vi "ArduinoLib.vi"() -> ()   [LabVIEW 2020]
uses:
  <vilib>/LabVIEW Interface for Arduino/Type Defs/Board Type.ctl
  <vilib>/LabVIEW Interface for Arduino/Type Defs/Connection Type.ctl
  <vilib>/LabVIEW Interface for Arduino/LabVIEW Interface for Arduino.lvlib
panel:
  in  "Connection Type (USB/Serial)":T1
  in  "Bytes Per Packet (15)":u32=15
  in  "milliseconds to wait":u32
  in  "Time Out (100 ms)":i32=100
  in  "Bytes To Read (0)":u8
  out "Read Buffer":string
  in  "stop":bool
  out "error out":errorcluster
  in  "error in (no error)":errorcluster
  in  "Board Type (Uno)":T2
  in  "Baud Rate (115200)":u32=115200
  in  "VISA resource":refnum<visa-resource-name>
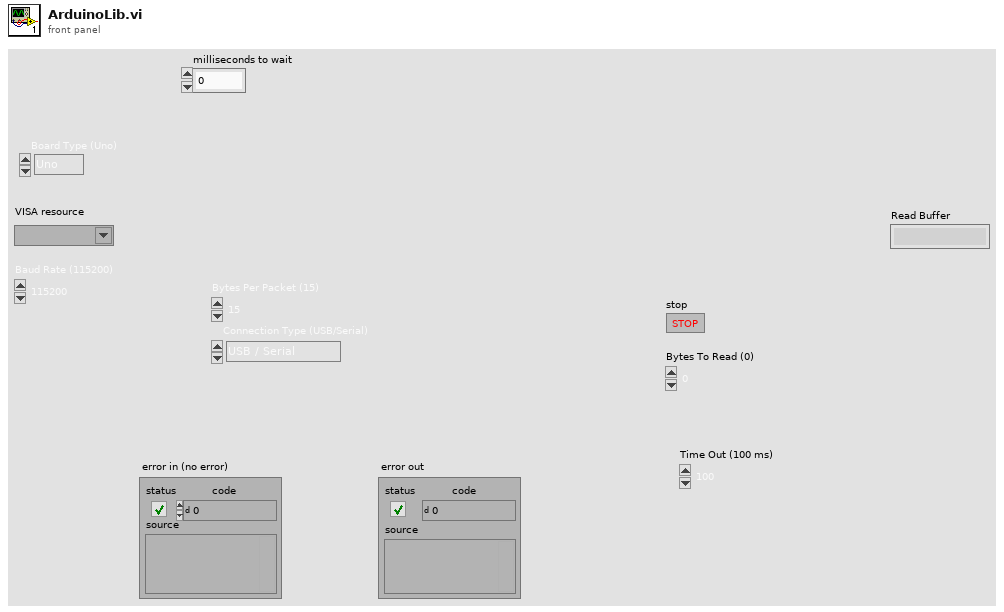
[diagram p1: front panel]
types:
  T1 = typedef "LabVIEW Interface for Arduino.lvlib/Connection Type.ctl" = enum8{"USB / Serial", "XBEE", "BlueSmirf (Bluetooth)"}
  T2 = typedef "LabVIEW Interface for Arduino.lvlib/Board Type.ctl" = enum16{"Uno", "Dimuelanove w/Atmega 328", "Mega 2560"}
  T3 = typedef "LabVIEW Interface for Arduino.lvlib/Arduino Resource.ctl" = cluster{"VISA resource":refnum<visa-resource-name>, "Board Type":T2, "Connection Type":enum8{"USB / Serial"}, "Bytes Per Packet (15)":u8}
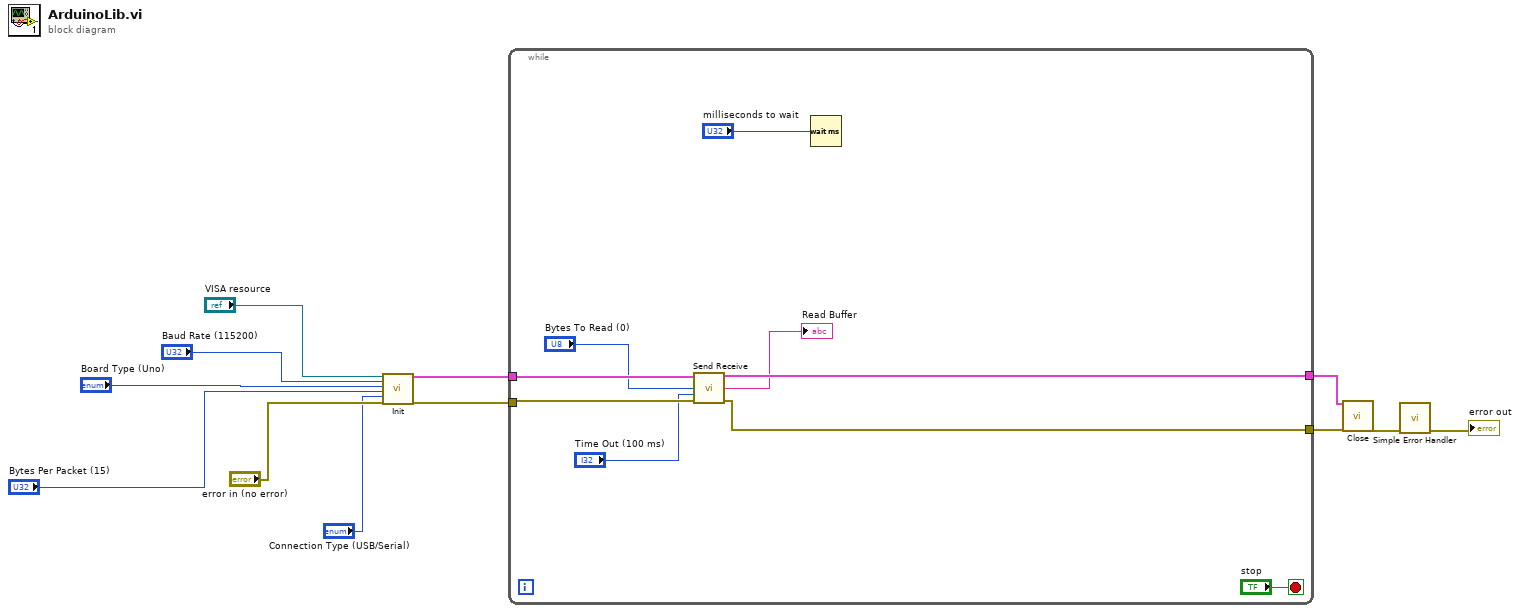
[diagram p0: block diagram]
diagram:
  n1 = call <vilib>:"Init.vi"("VISA resource"="VISA resource", "Baud Rate (115200)"="Baud Rate (115200)", "Board Type (Uno)"="Board Type (Uno)", "Bytes Per Packet (15)"="Bytes Per Packet (15)", "Connection Type (USB/Serial)"="Connection Type (USB/Serial)", "error in"="error in (no error)") -> ("Arduino Resource"=w8:T3, "error out"=w7:errorcluster)  [unwired: 12 in]
  n2 = while {
    tunnel: w8 -> [w19]
    tunnel: w7 -> [w20]
    tunnel: [w13] -> w4
    tunnel: [w18] -> w3
    stop <- "stop" stop-if-true
    n3 = call <vilib>:"Send Receive.vi"("Arduino Resource"=w19, "Bytes To Read (0)"="Bytes To Read (0)", "Time Out (100 ms)"="Time Out (100 ms)", "error in"=w20) -> ("Arduino Resource"=w18:T3, "Read Buffer"=→"Read Buffer":string, "error out"=w13:errorcluster)  [unwired: 9 in]
    n4 = Wait (ms)(milliseconds to wait="milliseconds to wait") -> ()  [unwired: 1 out]
  }
  n5 = call <vilib>:"Close.vi"("Arduino Resource"=w3, "error in"=w4) -> ("error out"=w6:errorcluster)  [unwired: 13 in]
  n6 = call <vilib>:"Simple Error Handler.vi"("error in (no error)"=w6) -> ("error out"=→"error out":errorcluster)  [unwired: 4 in, 4 out]
